vi "test Blob Lease.vi"(8 "error in (no error)":errorcluster, 11 "TestCase in":refnum<class "Test_Blob.lvclass">) -> (0 "error out":errorcluster, 3 "TestCase out":refnum<class "Test_Blob.lvclass">)   [LabVIEW 2015, in "Test_Blob.lvclass"]
uses:
  Test_Blob.lvclass
  Blob Storage/Blob Type.ctl
  Global Parameters.vi
  Core/Session/Session.lvclass
  Blob Storage/NI_Azure_Blob.lvlib
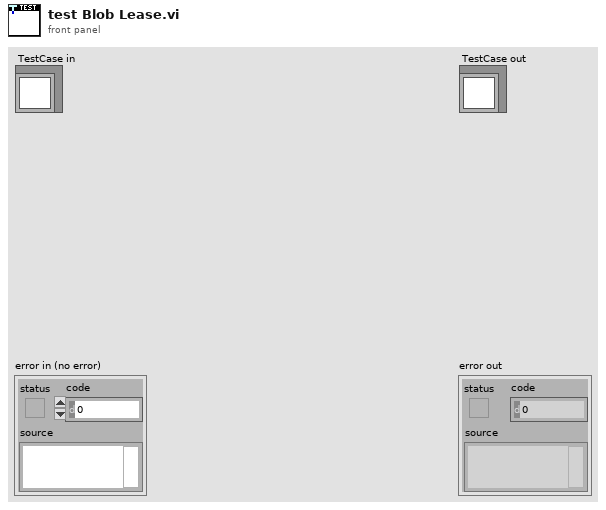
[diagram p1: front panel]
types:
  T1 = typedef "NI_Azure_Blob.lvlib/Blob Type.ctl" = enum16{"BlockBlob", "PageBlob", "AppendBlob"}
  T2 = typedef "NI_Azure_Core.lvlib/Session.lvclass/Azure Credentials.ctl" = cluster{"Storage Account Name":string, "Access Key":string}
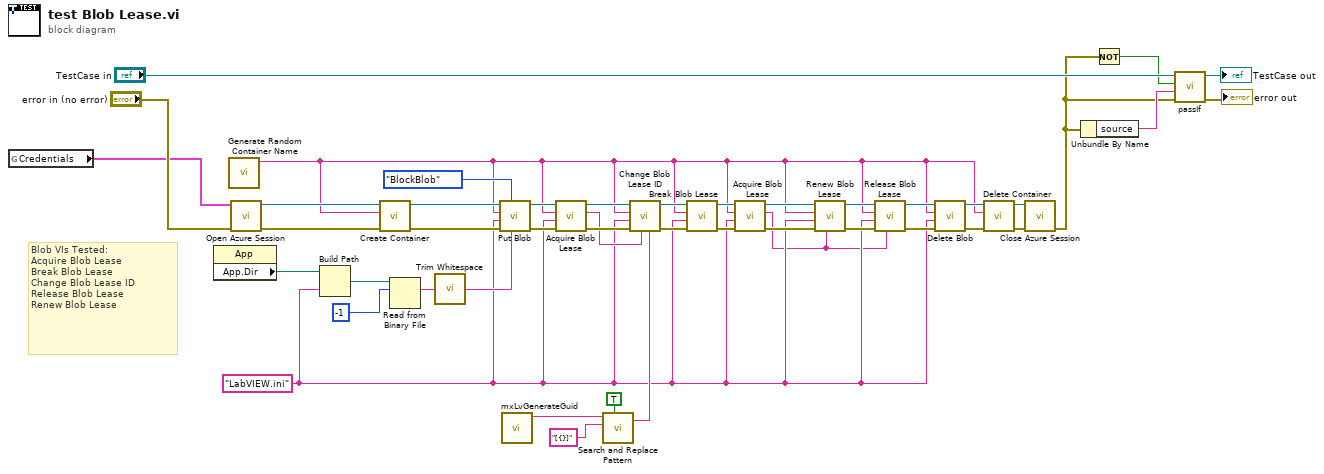
[diagram p0: block diagram]
diagram:
  w2 = "LabVIEW.ini"
  # "Blob VIs Tested:\nAcquire Blob Lease\nBreak Blob Lease\nChange Blob Lease ID\nRelease Blob Lease\nRenew Blob Lease"
  n1 = global read "Global Parameters.vi" "Credentials"() -> (w29:T2)
  n2 = property class="App"() -> ("App.Dir"=w40:path)  [unwired: 2 in, 2 out]
  n3 = call "Generate Random Container Name.vi"() -> ("Random Container Name"=w3:string)  [unwired: 11 in]
  n4 = call "Open Azure Session.vi"("error in (no error)"="error in (no error)", "Credentials"=w29) -> ("error out"=w30:errorcluster, "Azure Session"=w27:refnum<class "Session.lvclass">)  [unwired: 8 in]
  n5 = Build Path(base path=w40, name or relative path=w2) -> (appended path=w39:path)
  n6 = call "Create Container.vi"("error in (no error)"=w30, "Container"=w3, "Azure Session in"=w27) -> ("error out"=w37:errorcluster, "Azure Session out"=w36:refnum<class "Session.lvclass">)  [unwired: 7 in]
  n7 = Read from Binary File(10:-1 ("count (1)"), 11:w39) -> (2:w34:string)  [unwired: 4 in, 3 out]
  n8 = call <vilib>:"Trim Whitespace.vi"("string"=w34) -> ("trimmed string"=w26:string)  [unwired: 1 in]
  n9 = call "Put Blob.vi"("Blob Content"=w26, "Blob type"=Blob_Type."BlockBlob", "error in (no error)"=w37, "Blob"=w2, "Container"=w3, "Azure Session in"=w36) -> ("error out"=w35:errorcluster, "Azure Session out"=w22:refnum<class "Session.lvclass">)  [unwired: 4 in]
  n10 = call <resource>:"mxLvGenerateGuid.vi"() -> ("Value"=w16:string)  [unwired: 10 in, 1 out]
  n11 = call "Acquire Blob Lease.vi"("error in (no error)"=w35, "Blob"=w2, "Container"=w3, "Azure Session in"=w22) -> ("error out"=w23:errorcluster, "Lease ID"=w19:string, "Azure Session out"=w20:refnum<class "Session.lvclass">)  [unwired: 5 in]
  n12 = call <vilib>:"Search and Replace Pattern.vi"("string"=w16, "regular expression (\"\")"="[{}]" ("regular expression (\"\")"), "replace all? (F)"=TRUE) -> ("result string"=w7:string)  [unwired: 2 in, 1 out]
  n13 = call "Change Blob Lease ID.vi"("Proposed Lease ID"=w7, "Current Lease ID"=w19, "error in (no error)"=w23, "Blob"=w2, "Container"=w3, "Azure Session in"=w20) -> ("error out"=w21:errorcluster, "Azure Session out"=w12:refnum<class "Session.lvclass">)  [unwired: 4 in]
  n14 = call "Break Blob Lease.vi"("error in (no error)"=w21, "Blob"=w2, "Container"=w3, "Azure Session in"=w12) -> ("error out"=w13:errorcluster, "Azure Session out"=w5:refnum<class "Session.lvclass">)  [unwired: 6 in]
  n15 = call "Acquire Blob Lease.vi"("error in (no error)"=w13, "Blob"=w2, "Container"=w3, "Azure Session in"=w5) -> ("error out"=w6:errorcluster, "Lease ID"=w1:string, "Azure Session out"=w4:refnum<class "Session.lvclass">)  [unwired: 5 in]
  n16 = call "Renew Blob Lease.vi"("Lease ID"=w1, "error in (no error)"=w6, "Blob"=w2, "Container"=w3, "Azure Session in"=w4) -> ("error out"=w11:errorcluster, "Azure Session out"=w9:refnum<class "Session.lvclass">)  [unwired: 5 in]
  n17 = call "Release Blob Lease.vi"("Lease ID"=w1, "error in (no error)"=w11, "Blob"=w2, "Container"=w3, "Azure Session in"=w9) -> ("error out"=w10:errorcluster, "Azure Session out"=w8:refnum<class "Session.lvclass">)  [unwired: 5 in]
  n18 = call "Delete Blob.vi"("error in (no error)"=w10, "Blob"=w2, "Container"=w3, "Azure Session in"=w8) -> ("error out"=w33:errorcluster, "Azure Session out"=w32:refnum<class "Session.lvclass">)  [unwired: 6 in]
  n19 = call "Delete Container.vi"("error in (no error)"=w33, "Container"=w3, "Azure Session in"=w32) -> ("error out"=w28:errorcluster, "Azure Session out"=w24:refnum<class "Session.lvclass">)  [unwired: 7 in]
  n20 = call "Close Azure Session.vi"("error in (no error)"=w28, "Azure Session"=w24) -> ("error out"=w18:errorcluster)  [unwired: 9 in]
  n21 = Unbundle By Name(w18) -> ("source"=w41:string)
  n22 = Not(x=w18) -> (.not. x?=w17:bool)
  n23 = call-dynamic "passIf.vi"("error in (no error)"=w18, "message (\"\")"=w41, "pass"=w17, "TestCase in"="TestCase in") -> ("error out"=→"error out":errorcluster, "TestCase out"=→"TestCase out":refnum<class "Test_Blob.lvclass">)  [unwired: 6 in]
